vi "Rightable.vi"(1 "方块":dbl[][](array[numeric]), 2 "宽度":dbl, 3 "x":dbl) -> (0 "输出":bool)   [LabVIEW 2016]
panel:
  out "数值":dbl
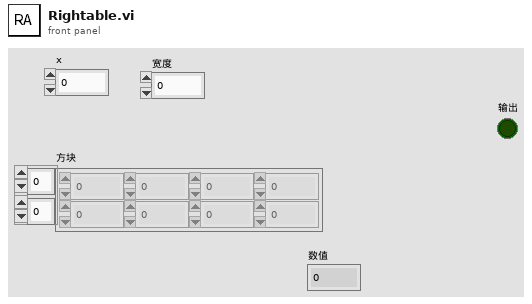
[diagram p1: front panel]
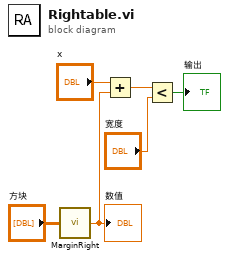
[diagram p0: block diagram]
diagram:
  n1 = call "MarginRight.vi"("输入"="方块") -> ("输出"=w4:dbl)
  "数值" <- w4
  n2 = Add(x="x", y=w4) -> (x+y=w3:dbl)
  n3 = Less?(x=w3, y="宽度") -> (x < y?=→"输出":bool)
